vi "Main.vi"() -> ()   [LabVIEW 2016]
doc: "The myRIO Project template acquires acceleration data from the onboard accelerometer and displays the changes of acceleration values in a waveform chart."
uses:
  <vilib>/myRIO/Instrument Drivers/Onboard IO/DIO/typedefs/DIO Reference.ctl
  <vilib>/myRIO/Common/Instrument Driver Framework/Utilities/typedefs/myRIO Generic Hardware Reference.ctl
  <vilib>/myRIO/Common/Instrument Driver Framework/Utilities/typedefs/Hardware Version Enum.ctl
  <vilib>/myRIO/Common/Instrument Driver Framework/Utilities/typedefs/myRIO v1.0 Reference.ctl
  <vilib>/myRIO/Common/Instrument Driver Framework/Utilities/typedefs/Generic FPGA Reference.ctl
  <vilib>/myRIO/Common/Instrument Driver Framework/myRIO v1.0/DIO/typedefs/DIO Channels List.ctl
  <vilib>/myRIO/Common/Instrument Driver Framework/myRIO v1.0/DIO/typedefs/DIO Channels Enum.ctl
  <vilib>/userdefined/High Color/nirio_resource_hc.ctl
  <vilib>/myRIO/Common/Instrument Driver Framework/Utilities/vis/Is FPGA Ref Available.vi
  <vilib>/myRIO/Common/Instrument Driver Framework/myRIO v1.0/DIO/vis/myRIO v1.1 Open DIO.vi
  <vilib>/myRIO/Instrument Drivers/Onboard IO/DIO/vis/Write.vi
  <vilib>/myRIO/Common/Instrument Driver Framework/Utilities/vis/Validate Channels.vi
  <vilib>/myRIO/Common/Instrument Driver Framework/myRIO v1.0/DIO/vis/myRIO v1.0 Reserve DIO.vi
  <vilib>/myRIO/Common/Instrument Driver Framework/myRIO v1.0/UART/vis/myRIO v1.0 Close UART.vi
  <vilib>/myRIO/Common/Instrument Driver Framework/myRIO v1.0/Resource Manager/vis/myRIO v1.0 Reserve Channel List.vi
  <vilib>/myRIO/Common/Instrument Driver Framework/myRIO v1.0/DIO/vis/myRIO v1.0 Build MUX Configuration DIO.vi
  <vilib>/myRIO/Common/Instrument Driver Framework/myRIO v1.0/Resource Manager/vis/myRIO v1.0 Reserve Channel.vi
  <vilib>/myRIO/Common/Instrument Driver Framework/myRIO v1.0/Resource Manager/vis/myRIO v1.0 Unreserve Channel.vi
  <vilib>/myRIO/Common/Instrument Driver Framework/myRIO v1.0/Resource Manager/vis/myRIO v1.0 Create Configuration List.vi
  <vilib>/myRIO/Common/Instrument Driver Framework/myRIO v1.0/Resource Manager/vis/myRIO v1.0 Build Mutex Name.vi
  <vilib>/National Instruments/IoT Education Toolkit Beta/TW API/TW_GetPropertyValues_Int.vi
  <vilib>/Utility/VariantDataType/GetNumericInfo.vi
  <vilib>/Utility/error.llb/Error Cluster From Error Code.vi
  <vilib>/myRIO/Common/Instrument Driver Framework/myRIO v1.0/myRIO v1.1 Open.vi
  <vilib>/myRIO/Common/Instrument Driver Framework/Utilities/vis/IO Manager.vi
  <vilib>/myRIO/Common/Instrument Driver Framework/Utilities/vis/Configuration Manager.vi
  <vilib>/myRIO/Common/Instrument Driver Framework/myRIO v1.0/Resource Manager/vis/myRIO v1.0 Configure IO.vi
  <vilib>/myRIO/Common/Instrument Driver Framework/myRIO v1.0/myRIO v1.0 Close.vi
  <vilib>/myRIO/Common/Instrument Driver Framework/myRIO v1.0/DIO/vis/myRIO v1.0 Write DIO.vi
  <vilib>/myRIO/Common/Instrument Driver Framework/Utilities/vis/FPGA Ref Manager.vi
  <vilib>/myRIO/Common/Instrument Driver Framework/myRIO v1.0/myRIO v1.0 Reset FPGA.vi
  <vilib>/myRIO/Common/Instrument Driver Framework/myRIO v1.0/IRQ/vis/myRIO v1.0 IRQ Info FGV.vi
  <vilib>/myRIO/Common/Instrument Driver Framework/myRIO v1.0/IRQ/vis/myRIO v1.0 Timer IRQ Info FGV.vi
  <vilib>/myRIO/Common/Instrument Driver Framework/myRIO v1.0/IRQ/vis/myRIO v1.0 ISR Agent.vi
  <vilib>/myRIO/Express VI/Onboard Devices/LED/LED Express VI.xnode
  <vilib>/myRIO/Instrument Drivers/Onboard IO/DIO/vis/myRIO DIO Open.xnode
  <vilib>/myRIO/Instrument Drivers/Utilities/Utilities.lvlib
  <vilib>/National Instruments/IoT Education Toolkit Beta/TW API/Thing.lvclass
  <vilib>/National Instruments/IoT Education Toolkit Beta/TW API/Properties.lvclass
  <vilib>/myRIO/Instrument Drivers/Onboard IO/DIO/DIO.lvlib
panel:
  in  "Stop":bool
  out "LED3":bool
  out "LED2":bool
  out "LED1":bool
  out "LED0":bool
  out "error out":errorcluster
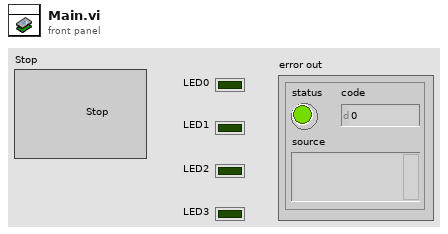
[diagram p1: front panel]
types:
  T1 = typedef "DIO.lvlib/DIO Reference.ctl" = cluster{"myRIO Reference":T2, "DIO Channels List":T6}
  T2 = typedef "myRIO Generic Hardware Reference.ctl" = cluster{"myRIO Model":T3, "myRIO Hardware Reference":T4}
  T3 = typedef "Hardware Version Enum.ctl" = enum16{"Unknown", "myRIO-1900", "myRIO-1950", "roboRIO", "NI ELVIS RIO CM"}
  T4 = typedef "myRIO v1.0 Reference.ctl" = cluster{"Generic FPGA Reference":T5, "Allow multiple opens":bool}
  T5 = typedef "Generic FPGA Reference.ctl" = refnum<k20>
  T6 = typedef "DIO Channels List.ctl" = T7[]
  T7 = typedef "DIO Channels Enum.ctl" = enum16{"Not Connected", "C/DIO0", "C/DIO1", "C/DIO2", "C/DIO3", "C/DIO4", "C/DIO5", "C/DIO6", "C/DIO7", "A/DIO0", "A/DIO1", "A/DIO2", "A/DIO3", "A/DIO4", "A/DIO5", "A/DIO6", "A/DIO7", "A/DIO8", "A/DIO9", "A/DIO10", "A/DIO11", "A/DIO12", "A/DIO13", "A/DIO14", "A/DIO15", "B/DIO0", "B/DIO1", "B/DIO2", "B/DIO3", "B/DIO4", "B/DIO5", "B/DIO6", "B/DIO7", "B/DIO8", "B/DIO9", "B/DIO10", "B/DIO11", "B/DIO12", "B/DIO13", "B/DIO14", "B/DIO15", "LED0", "LED1", "LED2", "LED3", "Button0", "DIO/DIO0", "DIO/DIO1", "DIO/DIO2", "DIO/DIO3", "DIO/DIO4", "DIO/DIO5", "DIO/DIO6", "DIO/DIO7", "DIO/DIO8", "DIO/DIO9", "SPI/CS0", "SPI/CS1", "SPI/CS2", "SPI/CS3", "LED RADIO (Green)", "LED RADIO (Red)", "LED COMM (Green)", "LED COMM (Red)", "LED MODE (Green)", "LED MODE (Red)"}
  T8 = typedef "nirio_resource_hc.ctl" = tag
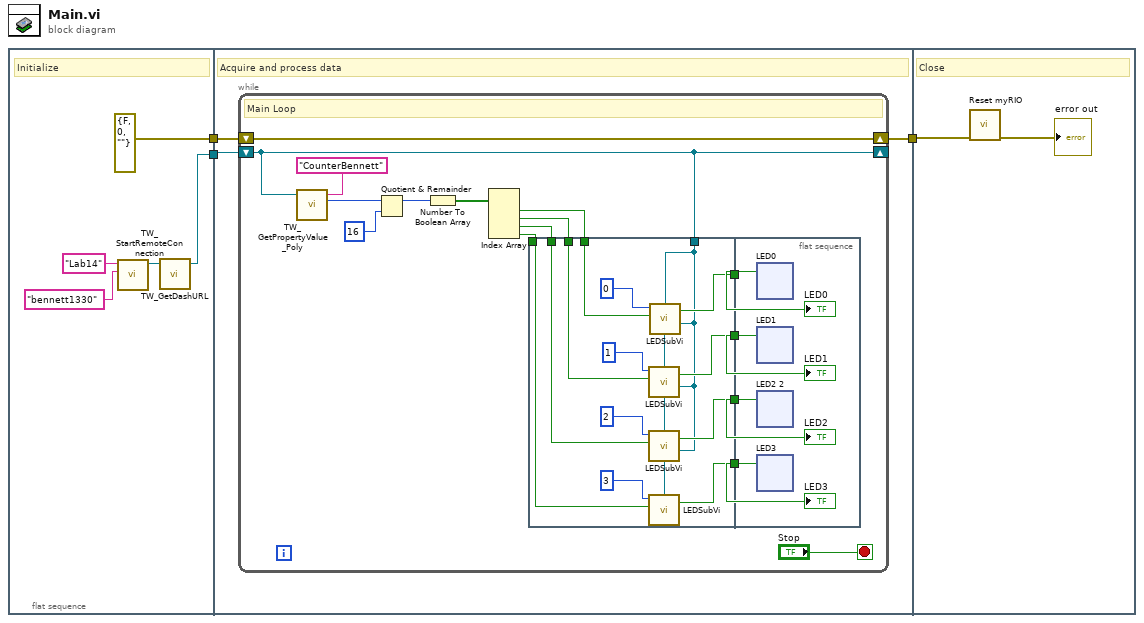
[diagram p0: block diagram]
diagram:
  n1 = flat-sequence {
    tunnel: [errorcluster {"status"=FALSE, "code"=0, "source"=""} ("error in (no error)")] -> w3
    tunnel: [w4] -> w1
    tunnel: w3 -> [w11]
    tunnel: [w10] -> w2
    tunnel: w1 -> [w9]
    tunnel: w2 -> [w186]
    frame #0 {
      # "Initialize"
      n2 = call <vilib>:"TW_StartRemoteConnection.vi"("Remote Username"="bennett1330", "Remote ThingName"="Lab14") -> ("Thing Out"=w5:refnum<class "Thing.lvclass">)  [unwired: 8 in, 1 out]
      n3 = call <vilib>:"TW_GetDashURL.vi"("Thing In"=w5) -> ("Thing Out"=w4:refnum<class "Thing.lvclass">)  [unwired: 4 in, 2 out]
    }
    frame #1 {
      # "Acquire and process data"
      n4 = while {
        shift-right: [w22] -> w10
        shift-left: w11 -> [w22]
        shift-right: [w12] -> _
        shift-left: w9 -> [w12]
        stop <- "Stop" stop-if-true
        # "Main Loop"
        n5 = call-poly <vilib>:"TW_GetPropertyValue_Poly.vi"("Thing in"=w12, "Property"="CounterBennett") -> ("value"=w26:i64)  [unwired: 3 in, 2 out]
        n6 = Quotient & Remainder(x=w26, y=i64 16) -> (x-y*floor(x/y)=w23:i64)  [unwired: 1 out]
        n7 = Number To Boolean Array(number=w23) -> (Boolean array=w24:bool[])
        n8 = Index Array(array=w24) -> (element #1=w20:bool, element #2=w19:bool, element #3=w18:bool, element #4=w17:bool)  [unwired: 4 in]
        n9 = flat-sequence {
          tunnel: w20 -> [w32]
          tunnel: w19 -> [w31]
          tunnel: w18 -> [w30]
          tunnel: w17 -> [w29]
          tunnel: [w36] -> w16
          tunnel: [w35] -> w15
          tunnel: [w34] -> w14
          tunnel: [w33] -> w13
          tunnel: w12 -> [w28]
          tunnel: w16 -> [w44]
          tunnel: w15 -> [w43]
          tunnel: w14 -> [w42]
          tunnel: w13 -> [w41]
          frame #0 {
            n10 = call "LEDSubVi.vi"("Thing in"=w28, "Numeric"=1, "ValueToWrite"=w31) -> ("WritenValue"=w35:bool)  [unwired: 6 in]
            n11 = call "LEDSubVi.vi"("Thing in"=w28, "Numeric"=2, "ValueToWrite"=w30) -> ("WritenValue"=w34:bool)  [unwired: 6 in]
            n12 = call "LEDSubVi.vi"("Thing in"=w28, "Numeric"=3, "ValueToWrite"=w29) -> ("WritenValue"=w33:bool)  [unwired: 6 in]
            n13 = call "LEDSubVi.vi"("Thing in"=w28, "Numeric"=0, "ValueToWrite"=w32) -> ("WritenValue"=w36:bool)  [unwired: 6 in]
          }
          frame #1 {
            n14 = xnode ("LED0")("LED0"=w44) -> ()  [unwired: 1 in, 1 out]
            n15 = xnode ("LED1")("LED1"=w43) -> ()  [unwired: 1 in, 1 out]
            n16 = xnode ("LED2 2")("LED2"=w42) -> ()  [unwired: 1 in, 1 out]
            n17 = xnode ("LED3")("LED3"=w41) -> ()  [unwired: 1 in, 1 out]
            "LED0" <- w44
            "LED1" <- w43
            "LED2" <- w42
            "LED3" <- w41
          }
        }
      }
    }
    frame #2 {
      # "Close"
      n18 = call <vilib>:"Reset myRIO.vi"("error in (no error)"=w186) -> ("error out"=→"error out":errorcluster)  [unwired: 10 in]
    }
  }
